vi "cs-scanning_altztrig.vi"() -> ()   [LabVIEW 2017]
uses:
  controls/boolean_info.ctl
  z-axis-params.ctl
  <vilib>/rvi/Emulation/niFpgaGetClockAttributes.vi
  <vilib>/rvi/Emulation/niFpgaSctlEmulationGetInTimedLoop.vi
  <vilib>/rvi/Emulation/niFpgaEmulationReportErrorSimple.vi
  <vilib>/rvi/Emulation/niFpgaProcessEmulError.vi
  <vilib>/rvi/eio/common/nirviEmuTemplateMethod_errors.vi
  <vilib>/rvi/Emulation/niFpgaEmulationIsFPGAContextNoSignature.vi
  <vilib>/rvi/DataTransferAndStorage/Container/Common/niFpgaContainerGetUniqueNameForEmu.vi
  <vilib>/rvi/Memory/Memory_Emulation/niFpgaMemoryEmulationCacheClearOnFirstRun.vi
  <vilib>/rvi/Memory/Memory_Emulation/nirvimemoryEmulationManagerCache_MakeExclusive.vi
  <vilib>/rvi/Memory/Memory_Emulation/niFpgaMemoryEmulationValidateCache.vi
  <vilib>/rvi/Memory/Memory_Emulation/nirvimemoryEmulationManagerCache_InsertValue.vi
  <vilib>/Utility/error.llb/Clear Errors.vi
  <vilib>/rvi/Memory/Memory_Emulation/nirvimemoryEmulationManagerCache_ReleaseExclusive.vi
  <vilib>/rvi/Memory/Memory_Emulation/nirvimemoryEmulationManagerCache_GetValue.vi
  <vilib>/rvi/Memory/Memory_Emulation/nirvimemoryEmulationManagerCache_SetValue.vi
  <vilib>/rvi/Emulation/niFpgaCriticalErrorInLSC.vi
  <vilib>/eio/EIONode/EIONode.xnode
  <vilib>/rvi/DataTransferAndStorage/Container/XNode/niFpgaContainer.xnode
  <vilib>/rvi/DataTransferAndStorage/Register/Emulation/niFpgaRegisterEmulation.vi
  FPGA-data-logging.lvlib
  libimaging-cs.lvlib
panel:
  in  "step_down_frac":fxp<+,8,1>
  out "state1-count":u64
  out "state5-count":u64
  out "state4-count":u64
  out "state3-count":u64
  out "state2-count":u64
  in  "collect all":bool
  in  "collect move":bool=TRUE
  out "iter":i32
  out "entity-index":i16
  out "All Done":bool
  in  "TsTicks":u32=1600
  in  "z-axis-params":T1={"TOL"=0.3, "ramp_rate"=0.0, "z_u_max"=5.0, "setpoint"=0.0, "Ki"=0.001, "Z_error_threshold"=0.0, "Z_settled_samples_threshold "=0, "z_UP"=0.0, "zup_N"=0, "TF Order"=2, "Num"=[-0.00254, 0.000408, 0.00295, 0.0, 0.0, 0.0, 0.0, 0.0, 0.0], "Den"=[0.982758, -1.98194, 1.0, 0.0, 0.0, 0.0, 0.0, 0.0, 0.0]} {"Z_error_threshold" format="%#_13g"; "ramp_rate" format="%#_13g"; "TOL" format="%#_13g"}
  out "number-settled-samples-Z":i16
  out "Current Case":i16
  out "boolean \nindicators":T2
  out "z-u(k)":sgl
  in  "ABORT":bool
  out "read fifo timeout":bool
  in  "numEntities":i16
  in  "init Z up":fxp<+/-,16,5>
  in  "trigger-0":bool
  out "number-settled-samples-y":i16
  out "number-settled-samples-x":i16
  in  "xy-error-threshold":sgl format="%#_13g"
  in  "settled-samples\nthreshold":i16
  in  "Ki-xy":sgl=0.001 format="%#_13g"
  in  "xy-bound":sgl
  in  "initial case":i16
  # "- If collect all = fasle and collect move = false,\nwe only collect measurement data.\n- If collect all = false, and collect move = true,\nwe collect measurement and move data.\n- If collect all = true, we collect everything."
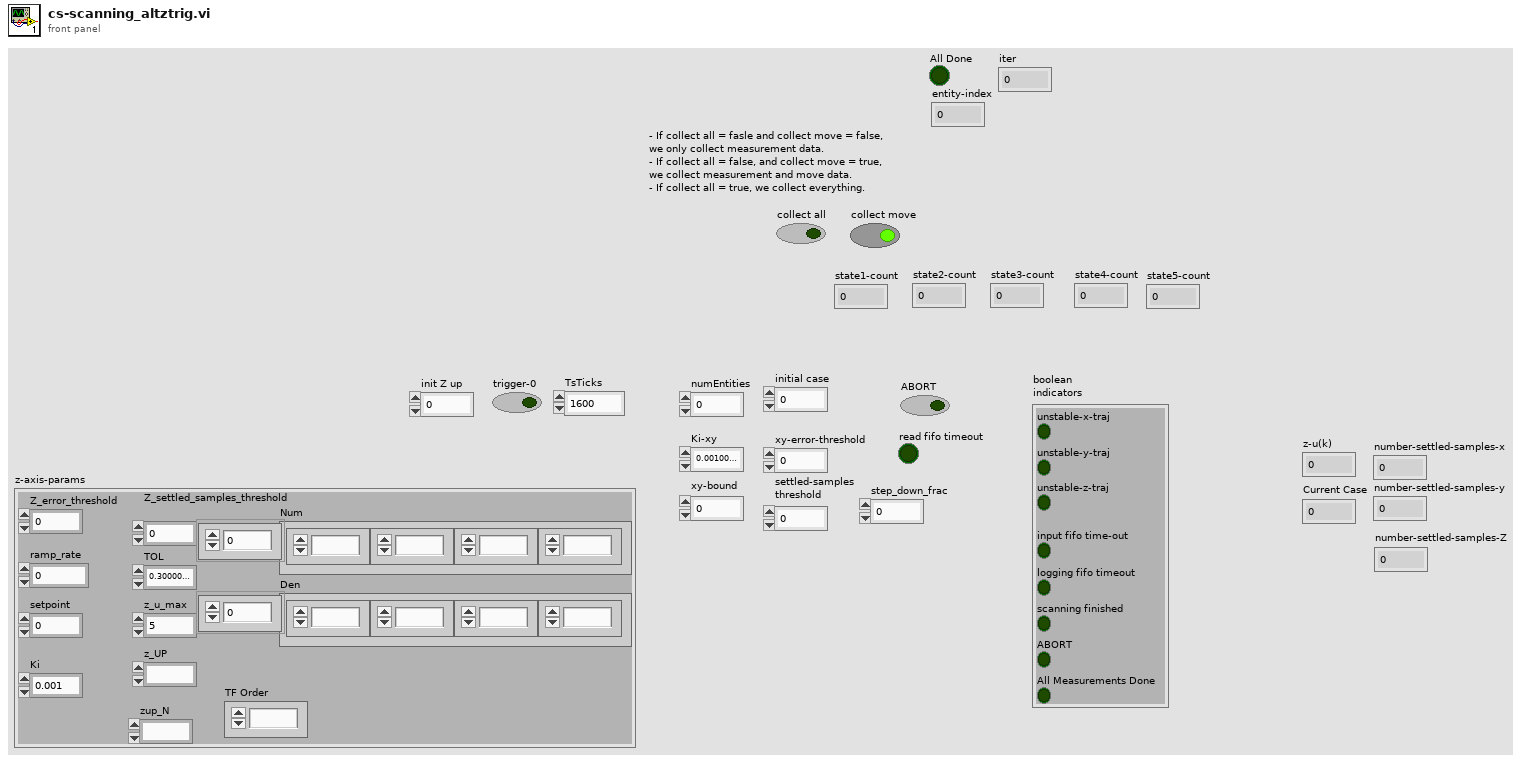
[diagram p1: front panel]
types:
  T1 = typedef "z-axis-params.ctl" = cluster{"TOL":sgl, "ramp_rate":sgl, "z_u_max":sgl, "setpoint":sgl, "Ki":sgl, "Z_error_threshold":sgl, "Z_settled_samples_threshold ":i16, "z_UP":fxp<+/-,16,5>, "zup_N":i16, "TF Order":i32, "Num":sgl[], "Den":sgl[]}
  T2 = typedef "boolean_info.ctl" = cluster{"unstable-z-traj":bool, "input fifo time-out":bool, "logging fifo timeout":bool, "scanning finished":bool, "unstable-x-traj":bool, "unstable-y-traj":bool, "ABORT":bool, "All Measurements Done":bool}
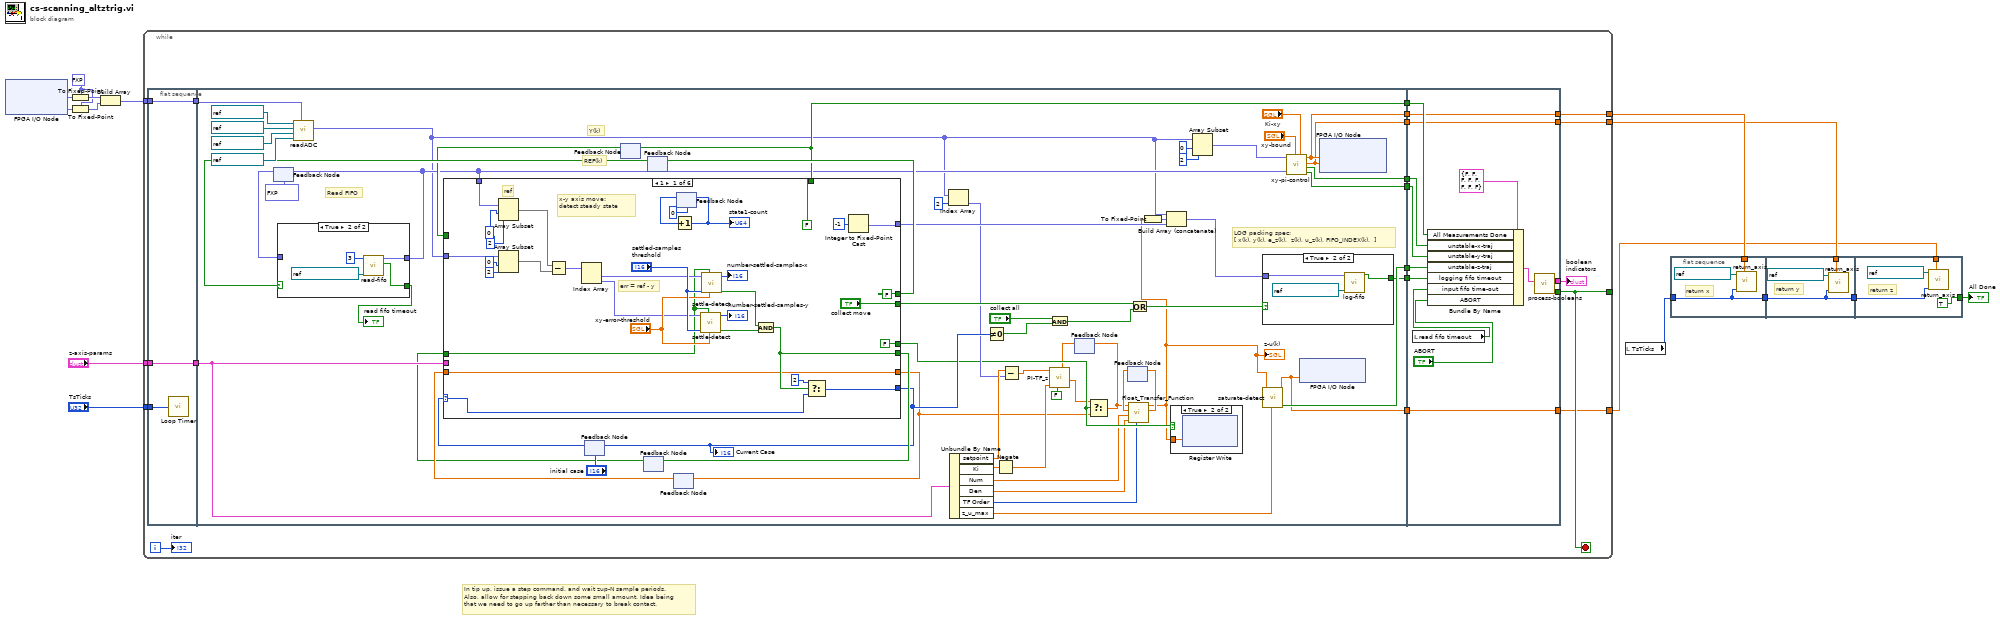
[diagram p0: block diagram]
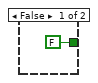
[diagram p3: hidden frame]
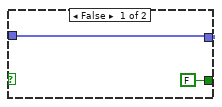
[diagram p4: hidden frame]
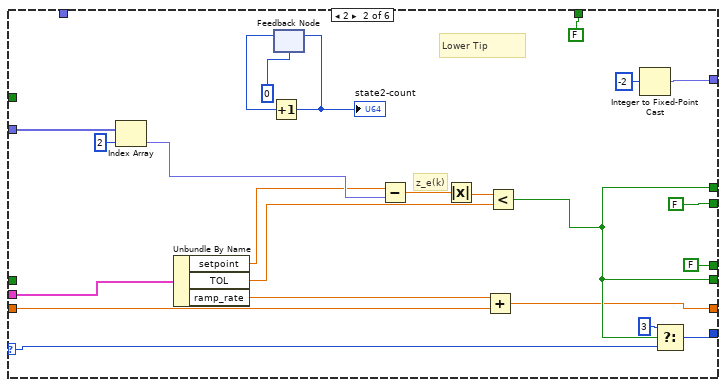
[diagram p5: hidden frame]
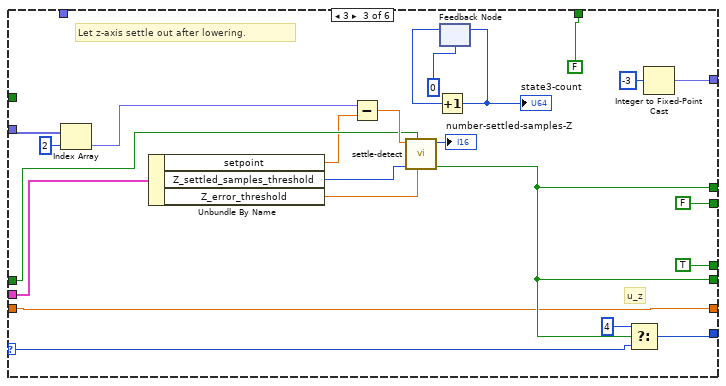
[diagram p6: hidden frame]
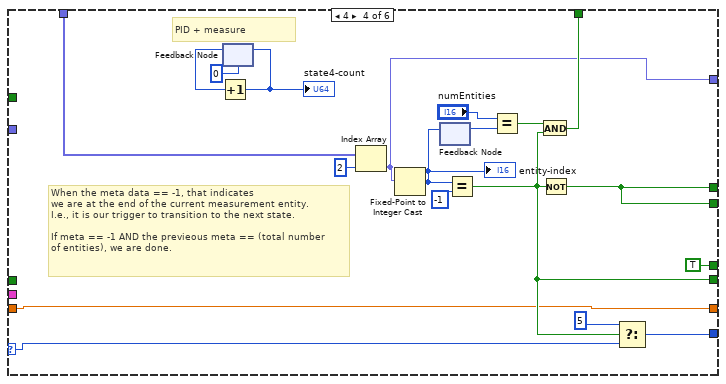
[diagram p7: hidden frame]
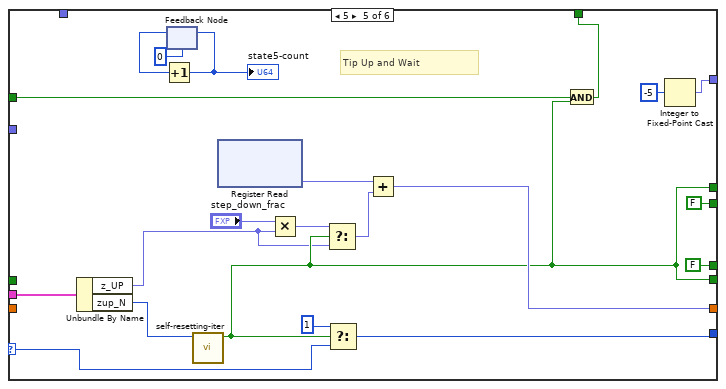
[diagram p8: hidden frame]
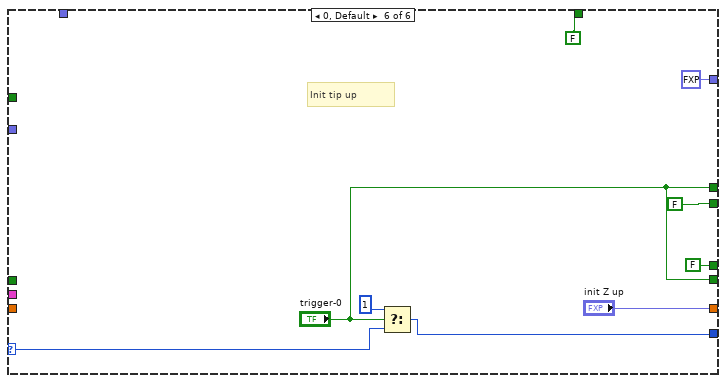
[diagram p9: hidden frame]
diagram:
  w10 = fxp<+/-,16,5> 0.0 ("fixed-point type")
  # "In tip up, issue a step command, and wait zup-N sample periods.\nAlso, allow for stepping back down some small amount. Idea being \nthat we need to go up farther than necessary to break contact."
  n1 = xnode "FPGA I/O Node"() -> ("Mod2/AI0"=w13:fxp<+/-,24,5>, "Mod2/AI1"=w11:fxp<+/-,24,5>)  [unwired: 2 in, 2 out]
  n2 = To Fixed-Point(fixed-point type=w10, number=w13) -> (fixed-point=w15:fxp<+/-,16,5>)
  n3 = To Fixed-Point(fixed-point type=w10, number=w11) -> (fixed-point=w12:fxp<+/-,16,5>)
  n4 = Build Array(w15, w12) -> (w14:fxp<+/-,16,5>[])
  n5 = while {
    tunnel: w14 -> [w27]
    tunnel: "z-axis-params" -> [w26]
    tunnel: "TsTicks" -> [w25]
    tunnel: [w23] -> _
    tunnel: [w21] -> w4
    tunnel: [w19] -> w3
    tunnel: [w17] -> w2
    i -> [w16]
    stop <- w23 stop-if-true
    n6 = flat-sequence {
      tunnel: w27 -> [w37]
      tunnel: [w37] -> w34
      tunnel: w25 -> [w35]
      tunnel: w26 -> [w36]
      tunnel: [w36] -> w33
      tunnel: w34 -> [w95]
      tunnel: w33 -> [w71]
      tunnel: [w82] -> w32
      tunnel: [w81] -> w31
      tunnel: [w80] -> w30
      tunnel: [w79] -> w29
      tunnel: [w59] -> w28
      tunnel: [w74] -> w22
      tunnel: [w73] -> w20
      tunnel: [w72] -> w18
      tunnel: w32 -> [w249]
      tunnel: w31 -> [w248]
      tunnel: w30 -> [w247]
      tunnel: w29 -> [w244]
      tunnel: w28 -> [w241]
      tunnel: [w240] -> w23
      tunnel: [w239] -> w24
      tunnel: w22 -> [w238]
      tunnel: [w238] -> w21
      tunnel: w20 -> [w237]
      tunnel: [w237] -> w19
      tunnel: [w236] -> w17
      tunnel: w18 -> [w236]
      frame #0 {
        n7 = call "Loop Timer"("Count(Ticks)"=w35) -> ()  [unwired: 1 out]
      }
      frame #1 {
        # "REF(k)"
        # "Y(k)"
        # "LOG packing spec:\n[ x(k), y(k), e_z(k),  z(k), u_z(k), FIFO_INDEX(k),  ]"
        # "Read FIFO"
        n8 = feedback #1(fxp<+/-,16,5>[] [0.0, 0.0, 0.0] ("unpacked-data")) -> (w86:fxp<+/-,16,5>[])
        n9 = call "readADC.vi"("x(0), y(0)"=w95, "z-height"=refnum<k21> "Mod2/AI3" ("y - ADC"), "z-err- ADC"=refnum<k21> "Mod2/AI2" ("y - ADC"), "y - ADC"=refnum<k21> "Mod2/AI1", "x - ADC"=refnum<k21> "Mod2/AI0") -> ("x_y_ze_z_k"=w54:fxp<+/-,17,6>[])  [unwired: 6 in]
        n10 = feedback #2("initial case") -> (w96:i16)
        n11 = feedback #3() -> (w70:bool)  [unwired: 1 in]
        n12 = feedback #4() -> (w68:bool)  [unwired: 1 in]
        n13 = feedback #5() -> (w76:bool)  [unwired: 1 in]
        n14 = case shown="True" w76 {
          tunnel: w86 -> [w104 _]
          tunnel: [w104 w106] -> w56
          tunnel: [FALSE ("timout?") w105] -> w78
          frame False {
          }
          frame True {
            n15 = call "read-fifo.vi"("FIFO In"=refnum<k21> "Host_to_FPGA", "numChan"=3) -> ("timout?"=w105:bool, "unpacked-data"=w106:fxp<+/-,16,5>[])  [unwired: 8 in]
          }
        }
        "read fifo timeout" <- w78
        n16 = feedback-in #1(w56) -> ()
        n17 = feedback #6() -> (w84:sgl)  [unwired: 1 in]
        n18 = case shown="1" w96 {
          selector: w96 -> [w132 w161 w179 w203 w225 w233]
          tunnel: ["collect move" FALSE FALSE ("trigger-0") w195 FALSE FALSE] -> w63
          tunnel: [w133 w156 w180 w204 w224 w235] -> w62
          tunnel: w54 -> [w127 w158 w184 _ _ _]
          tunnel: [FALSE w151 w173 w195 w210 "trigger-0"] -> w77
          tunnel: [w111 w146 w164 w187 w214 "init Z up"] -> w38
          tunnel: w84 -> [w111 w154 w164 w187 _ _]
          tunnel: w71 -> [_ w160 w177 _ w221 _]
          tunnel: [FALSE FALSE FALSE w194 w206 FALSE] -> w59
          tunnel: w56 -> [w122 _ _ w197 _ _]
          tunnel: w70 -> [_ _ _ _ w219 _]
          tunnel: w68 -> [w120 _ w168 _ _ _]
          tunnel: [w118 w151 w173 w193 w210 "trigger-0"] -> w69
          tunnel: [FALSE ("trigger-0") FALSE ("trigger-0") TRUE ("trigger-0") TRUE ("trigger-0") FALSE ("trigger-0") FALSE ("trigger-0")] -> w53
          tunnel: [w109 w142 w166 w188 w208 fxp<+/-,16,5> 0.0 ("Element")] -> w60
          frame 1 {
            # "err = ref - y"
            # "ref"
            # "x-y axis move: \ndetect steady state"
            n19 = Array Subset(array=w122, index=0, length=2) -> (w126:fxp<+/-,16,5>[])
            n20 = Array Subset(array=w127, index=0, length=2) -> (w125:fxp<+/-,17,6>[])
            n21 = Subtract(x=w126, y=w125) -> (x-y=w117:fxp<+/-,18,7>[])
            n22 = Index Array(array=w117) -> (element #1=w124:fxp<+/-,18,7>, element #2=w123:fxp<+/-,18,7>)  [unwired: 2 in]
            n23 = feedback #7(u64 0) -> (w114:u64)
            n24 = Increment(x=w114) -> (x+1=w115:u64)
            "state1-count" <- w115
            n25 = feedback-in #7(w115) -> ()
            n26 = call "settle-detect.vi"("error-max"="xy-error-threshold", "reset"=w120, "settled-samples\nthreshold"="settled-samples\nthreshold", "err(k)"=w123) -> ("has-settled"=w140:bool, "number-settled-samples"=→"number-settled-samples-y":u16)  [unwired: 6 in]
            n27 = call "settle-detect.vi"("error-max"="xy-error-threshold", "reset"=w120, "settled-samples\nthreshold"="settled-samples\nthreshold", "err(k)"=w124) -> ("has-settled"=w139:bool, "number-settled-samples"=→"number-settled-samples-x":u16)  [unwired: 6 in]
            n28 = And(x=w139, y=w140) -> (x .and. y?=w118:bool)
            n29 = Select(t=i16 2, s=w118, f=w132) -> (s? t:f=w133:i16)
            n30 = Integer to Fixed-Point Cast(integer=i16 -1) -> (fixed-point=w109:fxp<+/-,16,5>)  [unwired: 1 in]
          }
          frame 2 {
            # "z_e(k)"
            # "Lower Tip"
            n31 = Index Array(array=w158, index=2) -> (element=w157:fxp<+/-,17,6>)
            n32 = Unbundle By Name(w160) -> ("setpoint"=w145:sgl, "TOL"=w163:sgl, "ramp_rate"=w162:sgl)
            n33 = feedback #8(u64 0) -> (w149:u64)
            n34 = Increment(x=w149) -> (x+1=w150:u64)
            "state2-count" <- w150
            n35 = feedback-in #8(w150) -> ()
            n36 = Subtract(x=w145, y=w157) -> (x-y=w141:sgl)
            n37 = Absolute Value(x=w141) -> (abs(x)=w144:sgl)
            n38 = Add(x=w162, y=w154) -> (x+y=w146:sgl)
            n39 = Less?(x=w144, y=w163) -> (x < y?=w151:bool)
            n40 = Integer to Fixed-Point Cast(integer=i16 -2) -> (fixed-point=w142:fxp<+/-,16,5>)  [unwired: 1 in]
            n41 = Select(t=i16 3, s=w151, f=w161) -> (s? t:f=w156:i16)
          }
          frame 3 {
            # "u_z"
            # "Let z-axis settle out after lowering."
            n42 = Index Array(array=w184, index=2) -> (element=w182:fxp<+/-,17,6>)
            n43 = Unbundle By Name(w177) -> ("setpoint"=w165:sgl, "Z_settled_samples_threshold"=w176:i16, "Z_error_threshold"=w175:sgl)
            n44 = Subtract(x=w182, y=w165) -> (x-y=w185:sgl)
            n45 = call "settle-detect.vi"("error-max"=w175, "reset"=w168, "settled-samples\nthreshold"=w176, "err(k)"=w185) -> ("has-settled"=w173:bool, "number-settled-samples"=→"number-settled-samples-Z":u16)  [unwired: 6 in]
            n46 = feedback #9(u64 0) -> (w171:u64)
            n47 = Increment(x=w171) -> (x+1=w172:u64)
            "state3-count" <- w172
            n48 = feedback-in #9(w172) -> ()
            n49 = Select(t=i16 4, s=w173, f=w179) -> (s? t:f=w180:i16)
            n50 = Integer to Fixed-Point Cast(integer=i16 -3) -> (fixed-point=w166:fxp<+/-,16,5>)  [unwired: 1 in]
          }
          frame 4 {
            # "When the meta data == -1, that indicates\nwe are at the end of the current measurement entity.\nI.e., it is our trigger to transition to the next state.\n\nIf meta == -1 AND the previeous meta == (total number\nof entities), we are done."
            # "PID + measure"
            n51 = feedback #10(u64 0) -> (w191:u64)
            n52 = Increment(x=w191) -> (x+1=w192:u64)
            "state4-count" <- w192
            n53 = feedback-in #10(w192) -> ()
            n54 = Index Array(array=w197, index=2) -> (element=w188:fxp<+/-,16,5>)
            n55 = Fixed-Point to Integer Cast(1:w188) -> (0:w196:i16)
            "entity-index" <- w196
            n56 = feedback #11() -> (w198:i16)  [unwired: 1 in]
            n57 = feedback-in #11(w196) -> ()
            n58 = Equal?(x=w196, y=i16 -1) -> (x = y?=w193:bool)
            n59 = Equal?(x="numEntities", y=w198) -> (x = y?=w199:bool)
            n60 = And(x=w199, y=w193) -> (x .and. y?=w194:bool)
            n61 = Not(x=w193) -> (.not. x?=w195:bool)
            n62 = Select(t=i16 5, s=w193, f=w203) -> (s? t:f=w204:i16)
          }
          frame 5 {
            # "Tip Up and Wait"
            n63 = Unbundle By Name(w221) -> ("z_UP"=w209:fxp<+/-,16,5>, "zup_N"=w220:i16)
            n64 = feedback #12(u64 0) -> (w217:u64)
            n65 = Increment(x=w217) -> (x+1=w218:u64)
            "state5-count" <- w218
            n66 = feedback-in #12(w218) -> ()
            n67 = call "self-resetting-iter.vi"("N"=w220) -> ("Boolean"=w210:bool)  [unwired: 9 in, 1 out]
            n68 = xnode ("Register Read")() -> ("Data"=w222:fxp<+/-,16,5>)  [unwired: 1 in, 1 out]
            n69 = Multiply(x="step_down_frac", y=w209) -> (x*y=w213:fxp<+/-,24,6>)
            n70 = Select(t=w213, s=w210, f=w209) -> (s? t:f=w211:fxp<+/-,24,6>)
            n71 = Select(t=i16 1, s=w210, f=w225) -> (s? t:f=w224:i16)
            n72 = Add(x=w222, y=w211) -> (x+y=w214:fxp<+/-,25,7>)
            n73 = And(x=w219, y=w210) -> (x .and. y?=w206:bool)
            n74 = Integer to Fixed-Point Cast(integer=i16 -5) -> (fixed-point=w208:fxp<+/-,16,5>)  [unwired: 1 in]
          }
          frame 0, Default {
            # "Init tip up"
            n75 = Select(t=i16 1, s="trigger-0", f=w233) -> (s? t:f=w235:i16)
          }
        }
        "Current Case" <- w62
        n76 = feedback-in #2(w62) -> ()
        n77 = feedback-in #3(w59) -> ()
        n78 = feedback-in #4(w69) -> ()
        n79 = feedback-in #5(w77) -> ()
        n80 = feedback-in #6(w38) -> ()
        n81 = Index Array(array=w54, index=2) -> (element=w55:fxp<+/-,17,6>)
        n82 = Unbundle By Name(w71) -> ("setpoint"=w58:sgl, "Ki"=w45:sgl, "Num"=w52:sgl[], "Den"=w51:sgl[], "TF Order"=w49:i32, "z_u_max"=w50:sgl)
        n83 = Not Equal To 0?(x=w62) -> (x != 0?=w66:bool)
        n84 = Negate(x=w45) -> (-x=w44:sgl)
        n85 = Subtract(x=w58, y=w55) -> (x-y=w46:sgl)
        n86 = And(x="collect all", y=w66) -> (x .and. y?=w64:bool)
        n87 = feedback #13() -> (w40:sgl)  [unwired: 1 in]
        n88 = call "PI-TF_z.vi"("u(k-1)"=w40, "reset"=FALSE, "Ki"=w44, "e(k)"=w46) -> ("u(k)"=w42:sgl)  [unwired: 7 in]
        n89 = Select(t=w42, s=w53, f=w38) -> (s? t:f=w39:sgl)
        n90 = feedback-in #13(w39) -> ()
        n91 = feedback #14() -> (w47:sgl[])  [unwired: 1 in]
        n92 = call "Float_Transfer_Function.vi"("TF Order"=w49, "Den"=w51, "Num"=w52, "State In"=w47, "Input"=w39) -> ("State Out"=w48:sgl[], "Output"=w41:sgl)  [unwired: 4 in]
        "z-u(k)" <- w41
        n93 = feedback-in #14(w48) -> ()
        n94 = Or(x=w63, y=w64) -> (x .or. y?=w67:bool)
        n95 = To Fixed-Point(number=w41) -> (fixed-point=w61:fxp<+/-,16,5>)  [unwired: 1 in]
        n96 = Build Array (concatenate)(w54, w61, w60) -> (w83:fxp<+/-,17,6>[])
        n97 = case shown="True" w53 {
          tunnel: w41 -> [_ w98]
          frame False {
          }
          frame True {
            n98 = xnode ("Register Write")("Data"=w98) -> ()  [unwired: 1 in, 1 out]
          }
        }
        n99 = Array Subset(array=w54, index=0, length=2) -> (w85:fxp<+/-,17,6>[])
        n100 = case shown="True" w67 {
          tunnel: w83 -> [_ w101]
          tunnel: [FALSE ("logging-timeout?") w100] -> w79
          frame False {
          }
          frame True {
            n101 = call "log-fifo.vi"("FIFO In"=refnum<k21> "fpga-to-host2", "input-data"=w101) -> ("logging-timeout?"=w100:bool)  [unwired: 9 in]
          }
        }
        n102 = call "saturate-detect.vi"("bound"=w50, "x"=w41) -> ("saturated"=w80:bool, "sat(x)"=w72:sgl)  [unwired: 8 in]
        n103 = call "xy-pi-control.vi"("Ki-xy"="Ki-xy", "xy-umax"="xy-bound", "xy-ref"=w56, "x_k-y_k"=w85) -> ("u_y saturated"=w81:bool, "u_x saturated"=w82:bool, "sat(u_y)"=w73:sgl, "sat(u_x)"=w74:sgl)  [unwired: 4 in]
        n104 = xnode "FPGA I/O Node"("Mod1/AO2"=w72) -> ()  [unwired: 1 in, 1 out]
        n105 = xnode "FPGA I/O Node"("Mod1/AO0"=w74, "Mod1/AO1"=w73) -> ()  [unwired: 2 in, 2 out]
      }
      frame #2 {
        n106 = local read "read fifo timeout"() -> (w243:bool)
        n107 = Bundle By Name(cluster=T2 {"unstable-z-traj"=FALSE, "input fifo time-out"=FALSE, "logging fifo timeout"=FALSE, "scanning finished"=FALSE, "unstable-x-traj"=FALSE, "unstable-y-traj"=FALSE, "ABORT"=FALSE, "All Measurements Done"=FALSE} ("boolean errors"), "All Measurements Done"=w241, "unstable-x-traj"=w249, "unstable-y-traj"=w248, "unstable-z-traj"=w247, "logging fifo timeout"=w244, "input fifo time-out"=w243, "ABORT"="ABORT") -> (w245:T2)
        n108 = call "process-booleans.vi"("boolean indicators 2"=w245) -> ("scaning finished"=w240:bool, "boolean indicators"=w239:T2)  [unwired: 9 in]
      }
    }
    "boolean \nindicators" <- w24
    "iter" <- w16
  }
  n109 = local read "TsTicks"() -> (w5:u32)
  n110 = flat-sequence {
    tunnel: w5 -> [w251]
    tunnel: w4 -> [w252]
    tunnel: [w251] -> w7
    tunnel: w3 -> [w255]
    tunnel: w7 -> [w253]
    tunnel: [w253] -> w6
    tunnel: w2 -> [w259]
    tunnel: w6 -> [w257]
    tunnel: [TRUE] -> w1
    frame #0 {
      # "return x"
      n111 = call "return_axis.vi"("u(0)"=w252, "TsTicks"=w251, "FPGA I/O In"=refnum<k21> "Mod1/AO0") -> ()  [unwired: 9 in]
    }
    frame #1 {
      # "return y"
      n112 = call "return_axis.vi"("u(0)"=w255, "TsTicks"=w253, "FPGA I/O In"=refnum<k21> "Mod1/AO1") -> ()  [unwired: 9 in]
    }
    frame #2 {
      # "return z"
      n113 = call "return_axis.vi"("u(0)"=w259, "TsTicks"=w257, "FPGA I/O In"=refnum<k21> "Mod1/AO2") -> ()  [unwired: 9 in]
    }
  }
  "All Done" <- w1
